vi "Event Log.vi"(0 "Event log message":string, 7 "Priority":T1, 11 "error in (no error)":errorcluster, 12 "Disconnecting":bool) -> (15 "error out":errorcluster)   [LabVIEW 2011]
uses:
  Event Log - Priority.ctl
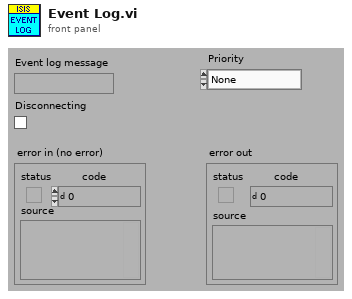
[diagram p1: front panel]
types:
  T1 = typedef "Event Log - Priority.ctl" = enum16{"None", "Log", "SECI and Log"}
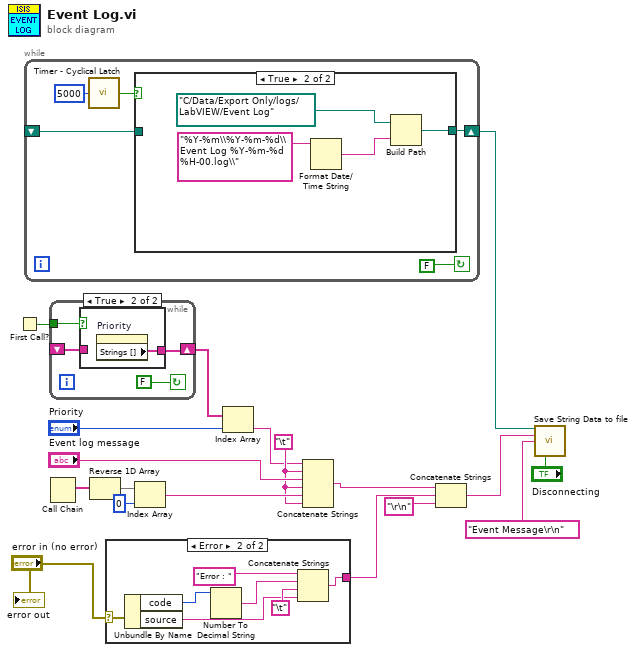
[diagram p0: block diagram]
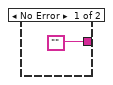
[diagram p3: hidden frame]
diagram:
  w4 = "\t"
  n1 = First Call?() -> (First Call?: T/F=w5:bool)
  n2 = while {
    shift-right: [w23] -> w16
    shift-left: _ -> [w20]
    stop <- FALSE continue-if-true
    n3 = call "Timer - Cyclical Latch.vi"("Timer (msec)"=u32 5000) -> ("Timer Trigger"=w21:bool)  [unwired: 14 in]
    n4 = case shown="True" w21 {
      tunnel: [w24 w25] -> w23
      tunnel: w20 -> [w24 _]
      frame False {
      }
      frame True {
        n5 = Format Date/Time String(time format string (%c)="%Y-%m\\%Y-%m-%d\\Event Log %Y-%m-%d %H-00.log\\") -> (date/time string=w26:string)  [unwired: 2 in]
        n6 = Build Path(base path=path "C:/Data/Export Only/logs/LabVIEW/Event Log", name or relative path=w26) -> (appended path=w25:path)
      }
    }
  }
  n7 = Call Chain() -> (call chain=w7:string[])
  n8 = while {
    tunnel: w5 -> [w32]
    shift-right: [w30] -> w3
    shift-left: _ -> [w31]
    stop <- FALSE continue-if-true
    n9 = case shown="True" w32 {
      tunnel: w31 -> [w33 _]
      tunnel: [w33 w34] -> w30
      frame False {
      }
      frame True {
        n10 = property on="Priority" class="Enum (strict)"() -> ("Strings []"=w34:string[])  [unwired: 2 in, 2 out]
      }
    }
  }
  n11 = Reverse 1D Array(array=w7) -> (reversed array=w6:string[])
  n12 = case shown="Error" "error in (no error)" {
    selector: "error in (no error)" -> [_ w42]
    tunnel: ["" w41] -> w11
    frame No Error {
    }
    frame Error {
      n13 = Unbundle By Name(w42) -> ("code"=w37:i32, "source"=w38:string)
      n14 = Number To Decimal String(number=w37) -> (decimal integer string=w36:string)  [unwired: 1 in]
      n15 = Concatenate Strings("Error : ", w36, "\t", w38) -> (w41:string)
    }
  }
  n16 = Index Array(array=w6, index=0) -> (element=w8:string)
  n17 = Index Array(array=w3, index="Priority") -> (element=w1:string)
  n18 = Concatenate Strings(w1, w4, "Event log message", w4, w8, w4) -> (w14:string)
  n19 = Concatenate Strings(w14, w11, "\r\n") -> (w13:string)
  n20 = call "Save String Data to file.vi"("Path"=w16, "String to save"=w13, "Header"="Event Message\r\n", "Disconnecting"="Disconnecting") -> ()  [unwired: 12 in]
  "error out" <- "error in (no error)"
